vi "Correlation Test.vi"(6 "alternative hypothesis":i32(ring) items=["r != 0"=0, "r > 0"=1, "r < 0"=-1], 8 "significance level":dbl=0.05 format="%.4g", 9 "type":enum32{"Pearson", "Spearman", "Kendall"}(ring), 10 "sample set y":dbl[](array[numeric]), 11 "sample set x":dbl[](array[numeric])) -> (0 "error":i32, 1 "rsig":dbl, 2 "p value":dbl=0.05 format="%.6g", 3 "reject null hypothesis":bool, 4 "correlation coefficient r":dbl)   [LabVIEW 2017, in "NI_Gmath.lvlib"]
doc: "Tests hypotheses about the association between two variables x and y."
uses:
  NI_Gmath.lvlib
panel:
  # "Correlation Test\nPearson, Spearman, Kendall"
  # ">="
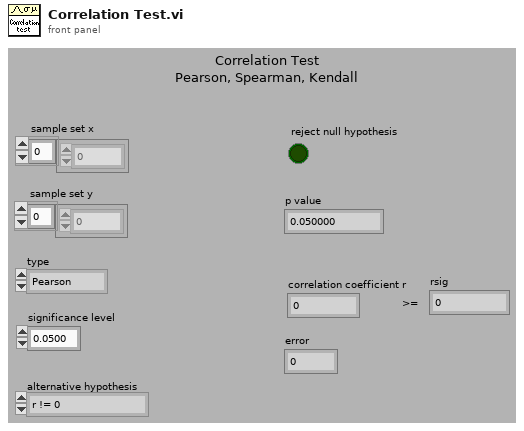
[diagram p1: front panel]
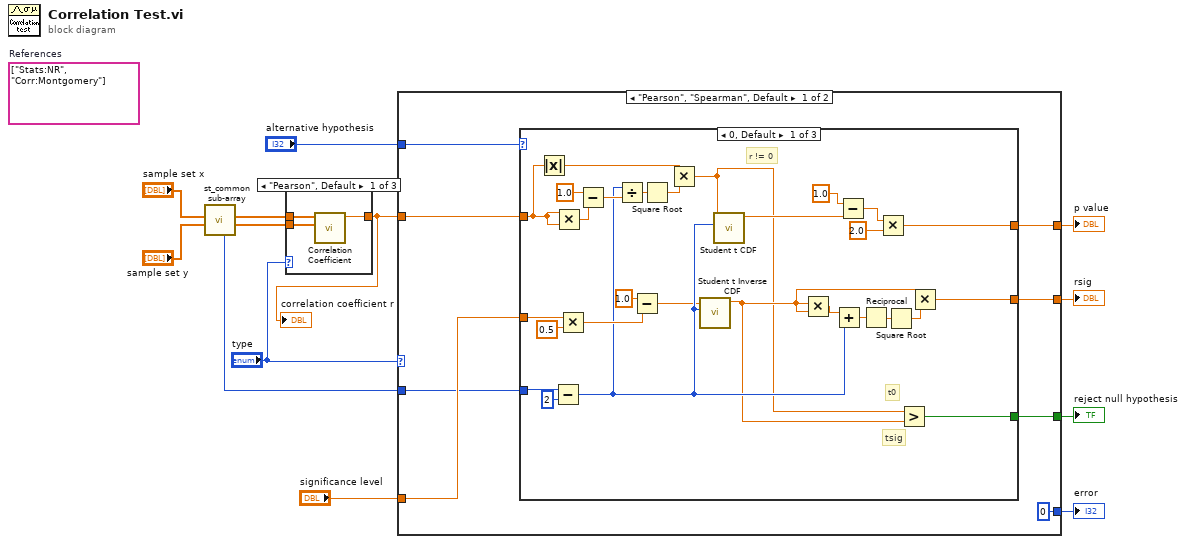
[diagram p0: block diagram]
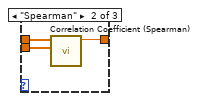
[diagram p2: hidden frame]
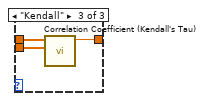
[diagram p3: hidden frame]
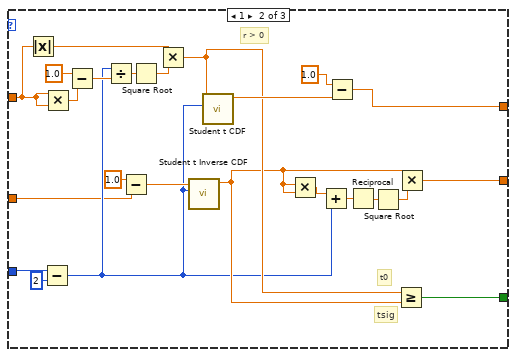
[diagram p4: hidden frame]
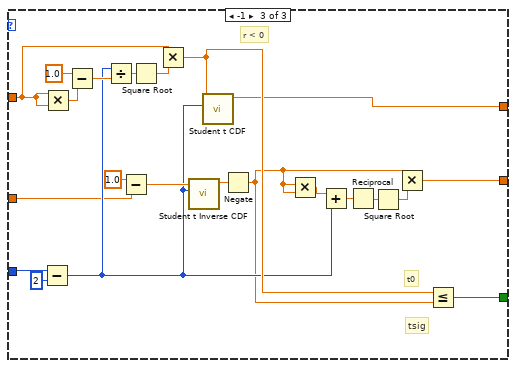
[diagram p5: hidden frame]
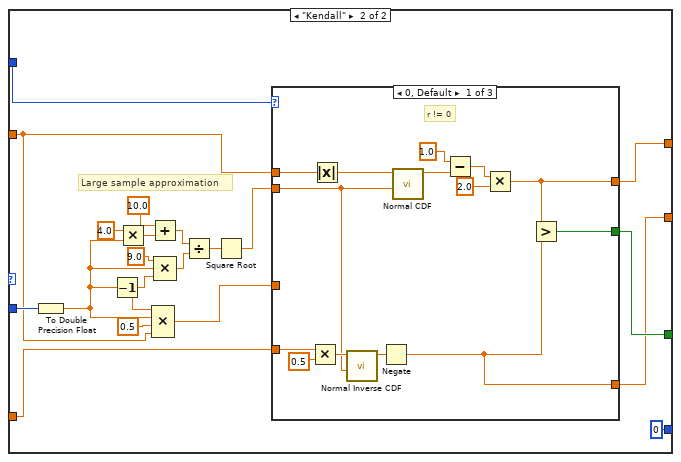
[diagram p6: hidden frame]
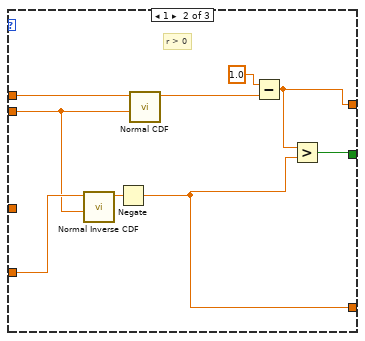
[diagram p7: hidden frame]
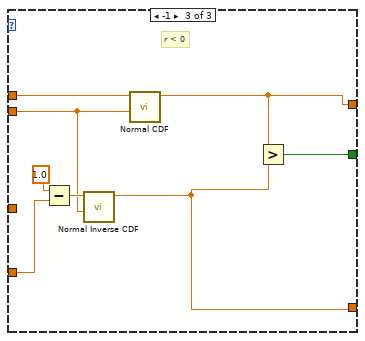
[diagram p8: hidden frame]
diagram:
  (unwired) string[] ["Stats:NR", "Corr:Montgomery"]  # References
  n1 = call "st_common sub-array.vi"(9:"array 1 in"="sample set y", 10:"array 1 in"="sample set x") -> (1:"array 1 out"=w11:dbl[], 2:"array 1 out"=w12:dbl[], "size"=w10:i32)  [unwired: 7 in]
  n2 = case shown="\"Pearson\", Default" "type" {
    tunnel: w12 -> [w16 w19 w22]
    tunnel: w11 -> [w15 w18 w21]
    tunnel: [w14 w17 w20] -> w9
    frame "Pearson", Default {
      n3 = call "Correlation Coefficient.vi"("Y"=w15, "X"=w16) -> ("correlation coefficient r"=w14:dbl)  [unwired: 8 in, 1 out]
    }
    frame "Spearman" {
      n4 = call "Correlation Coefficient (Spearman).vi"("Y"=w18, "X"=w19) -> ("correlation coefficient r"=w17:dbl)  [unwired: 8 in, 1 out]
    }
    frame "Kendall" {
      n5 = call "Correlation Coefficient (Kendall's Tau).vi"("Y"=w21, "X"=w22) -> ("correlation coefficient r"=w20:dbl)  [unwired: 8 in, 1 out]
    }
  }
  "correlation coefficient r" <- w9
  n6 = case shown="\"Pearson\", \"Spearman\", Default" "type" {
    tunnel: "significance level" -> [w30 w118]
    tunnel: w10 -> [w29 w113]
    tunnel: w9 -> [w28 w109]
    tunnel: [w27 w116] -> w8
    tunnel: [w26 w115] -> w6
    tunnel: "alternative hypothesis" -> [w25 w117]
    tunnel: [w24 w107] -> w2
    tunnel: [0 0] -> w1
    frame "Pearson", "Spearman", Default {
      n7 = case shown="0, Default" w25 {
        tunnel: w30 -> [w33 w59 w86]
        tunnel: w29 -> [w51 w79 w103]
        tunnel: [w42 w71 w96] -> w27
        tunnel: w28 -> [w41 w70 w85]
        tunnel: [w53 w60 w83] -> w26
        tunnel: [w34 w63 w89] -> w24
        frame 0, Default {
          # "tsig"
          # "t0"
          # "r != 0"
          n8 = Absolute Value(x=w41) -> (abs(x)=w45:dbl)
          n9 = Subtract(x=w51, y=2 ("x")) -> (x-y=w39:i32)
          n10 = Multiply(x=w41, y=w41) -> (x*y=w49:dbl)
          n11 = Multiply(x=w33, y=0.5) -> (x*y=w43:dbl)
          n12 = Subtract(x=1.0, y=w49) -> (x-y=w48:dbl)
          n13 = Divide(x=w39, y=w48) -> (x/y=w47:dbl)
          n14 = Subtract(x=1.0, y=w43) -> (x-y=w32:dbl)
          n15 = Square Root(x=w47) -> (sqrt(x)=w46:dbl)
          n16 = Multiply(x=w45, y=w46) -> (x*y=w31:dbl)
          n17 = call "Student t Inverse CDF.vi"("k degrees of freedom"=w39, "cdf(x)"=w32) -> ("x"=w36:dbl)  [unwired: 8 in, 1 out]
          n18 = call "Student t CDF.vi"("k degrees of freedom"=w39, "x"=w31) -> ("cdf(x)"=w56:dbl)  [unwired: 7 in, 2 out]
          n19 = Multiply(x=w36, y=w36) -> (x*y=w40:dbl)
          n20 = Add(x=w40, y=w39) -> (x+y=w38:dbl)
          n21 = Subtract(x=1.0, y=w56) -> (x-y=w54:dbl)
          n22 = Reciprocal(x=w38) -> (1/x=w37:dbl)
          n23 = Multiply(x=w54, y=2.0) -> (x*y=w53:dbl)
          n24 = Square Root(x=w37) -> (sqrt(x)=w35:dbl)
          n25 = Greater?(x=w31, y=w36) -> (0:w42:bool)
          n26 = Multiply(x=w36, y=w35) -> (x*y=w34:dbl)
        }
        frame 1 {
          # "tsig"
          # "t0"
          # "r > 0"
          n27 = Absolute Value(x=w70) -> (abs(x)=w73:dbl)
          n28 = Subtract(x=w79, y=2 ("x")) -> (x-y=w61:i32)
          n29 = Multiply(x=w70, y=w70) -> (x*y=w77:dbl)
          n30 = Subtract(x=1.0, y=w77) -> (x-y=w76:dbl)
          n31 = Divide(x=w61, y=w76) -> (x/y=w75:dbl)
          n32 = Subtract(x=1.0, y=w59) -> (x-y=w69:dbl)
          n33 = Square Root(x=w75) -> (sqrt(x)=w74:dbl)
          n34 = Multiply(x=w73, y=w74) -> (x*y=w68:dbl)
          n35 = call "Student t Inverse CDF.vi"("k degrees of freedom"=w61, "cdf(x)"=w69) -> ("x"=w62:dbl)  [unwired: 8 in, 1 out]
          n36 = call "Student t CDF.vi"("k degrees of freedom"=w61, "x"=w68) -> ("cdf(x)"=w81:dbl)  [unwired: 7 in, 2 out]
          n37 = Multiply(x=w62, y=w62) -> (x*y=w67:dbl)
          n38 = Add(x=w67, y=w61) -> (x+y=w66:dbl)
          n39 = Subtract(x=1.0, y=w81) -> (x-y=w60:dbl)
          n40 = Reciprocal(x=w66) -> (1/x=w65:dbl)
          n41 = Square Root(x=w65) -> (sqrt(x)=w64:dbl)
          n42 = Greater Or Equal?(x=w68, y=w62) -> (x >= y?=w71:bool)
          n43 = Multiply(x=w62, y=w64) -> (x*y=w63:dbl)
        }
        frame -1 {
          # "tsig"
          # "t0"
          # "r < 0"
          n44 = Subtract(x=w103, y=2 ("x")) -> (x-y=w87:i32)
          n45 = Multiply(x=w85, y=w85) -> (x*y=w101:dbl)
          n46 = Subtract(x=1.0, y=w101) -> (x-y=w100:dbl)
          n47 = Divide(x=w87, y=w100) -> (x/y=w99:dbl)
          n48 = Subtract(x=1.0, y=w86) -> (x-y=w95:dbl)
          n49 = Square Root(x=w99) -> (sqrt(x)=w98:dbl)
          n50 = Multiply(x=w85, y=w98) -> (x*y=w94:dbl)
          n51 = call "Student t Inverse CDF.vi"("k degrees of freedom"=w87, "cdf(x)"=w95) -> ("x"=w88:dbl)  [unwired: 8 in, 1 out]
          n52 = call "Student t CDF.vi"("k degrees of freedom"=w87, "x"=w94) -> ("cdf(x)"=w83:dbl)  [unwired: 7 in, 2 out]
          n53 = Negate(x=w88) -> (-x=w84:dbl)
          n54 = Multiply(x=w84, y=w84) -> (x*y=w93:dbl)
          n55 = Add(x=w93, y=w87) -> (x+y=w92:dbl)
          n56 = Reciprocal(x=w92) -> (1/x=w91:dbl)
          n57 = Square Root(x=w91) -> (sqrt(x)=w90:dbl)
          n58 = Multiply(x=w84, y=w90) -> (x*y=w89:dbl)
          n59 = Less Or Equal?(x=w94, y=w84) -> (x <= y?=w96:bool)
        }
      }
    }
    frame "Kendall" {
      # "Large sample approximation"
      n60 = To Double Precision Float(number=w113) -> (double precision float=w111:dbl)
      n61 = Decrement(x=w111) -> (x-1=w112:dbl)
      n62 = Multiply(x=4.0, y=w111) -> (x*y=w123:dbl)
      n63 = Add(x=10.0, y=w123) -> (x+y=w120:dbl)
      n64 = Compound Arithmetic op=MULTIPLY(w112, w111, 0.5 ("x"), w109) -> (w108:dbl)
      n65 = Compound Arithmetic op=MULTIPLY(9.0 ("x"), w111, w112) -> (w119:dbl)
      n66 = Divide(x=w120, y=w119) -> (x/y=w114:dbl)
      n67 = Square Root(x=w114) -> (sqrt(x)=w106:dbl)
      n68 = case shown="0, Default" w117 {
        tunnel: w118 -> [w137 w145 w154]
        tunnel: w109 -> [w134 w139 w152]
        tunnel: [w128 w143 w151] -> w115
        tunnel: [w125 w140 w148] -> w107
        tunnel: [w127 w142 w150] -> w116
        tunnel: w106 -> [w126 w141 w149]
        tunnel: w108 -> [_ _ _]
        frame 0, Default {
          # "r != 0"
          n69 = Multiply(x=w137, y=0.5) -> (x*y=w135:dbl)
          n70 = Absolute Value(x=w134) -> (abs(x)=w129:dbl)
          n71 = call "Normal Inverse CDF.vi"("std"=w126, "cdf(x)"=w135) -> ("x"=w136:dbl)  [unwired: 8 in, 1 out]
          n72 = Negate(x=w136) -> (-x=w125:dbl)
          n73 = call "Normal CDF.vi"("std"=w126, "x"=w129) -> ("cdf(x)"=w132:dbl)  [unwired: 8 in, 1 out]
          n74 = Subtract(x=1.0, y=w132) -> (x-y=w130:dbl)
          n75 = Multiply(x=w130, y=2.0) -> (x*y=w128:dbl)
          n76 = Greater?(x=w128, y=w125) -> (0:w127:bool)
        }
        frame 1 {
          # "r > 0"
          n77 = call "Normal Inverse CDF.vi"("std"=w141, "cdf(x)"=w145) -> ("x"=w144:dbl)  [unwired: 8 in, 1 out]
          n78 = Negate(x=w144) -> (-x=w140:dbl)
          n79 = call "Normal CDF.vi"("std"=w141, "x"=w139) -> ("cdf(x)"=w146:dbl)  [unwired: 8 in, 1 out]
          n80 = Subtract(x=1.0, y=w146) -> (x-y=w143:dbl)
          n81 = Greater?(x=w143, y=w140) -> (0:w142:bool)
        }
        frame -1 {
          # "r < 0"
          n82 = Subtract(x=1.0, y=w154) -> (x-y=w153:dbl)
          n83 = call "Normal Inverse CDF.vi"("std"=w149, "cdf(x)"=w153) -> ("x"=w148:dbl)  [unwired: 8 in, 1 out]
          n84 = call "Normal CDF.vi"("std"=w149, "x"=w152) -> ("cdf(x)"=w151:dbl)  [unwired: 8 in, 1 out]
          n85 = Greater?(x=w151, y=w148) -> (0:w150:bool)
        }
      }
    }
  }
  "error" <- w1
  "reject null hypothesis" <- w8
  "p value" <- w6
  "rsig" <- w2
